vi "Create Wheel Angular Velocity Row_Frame.vi"(7 "use zeros (F)":bool, 8 "error in (no error)":errorcluster, 10 "steering angle (rad)":dbl, 11 "wheel in":refnum<class "NI_Robotics_Wheel.lvclass">) -> (0 "error out":errorcluster, 2 "wheel angular velocity row":dbl[](array[numeric]), 3 "wheel out":refnum<class "NI_Robotics_Wheel.lvclass">)   [LabVIEW 2017, in "NI_Robotics_Wheel.lvclass"]
uses:
  <vilib>/robotics/Steering/Wheel/NI_Robotics_Wheel.lvclass
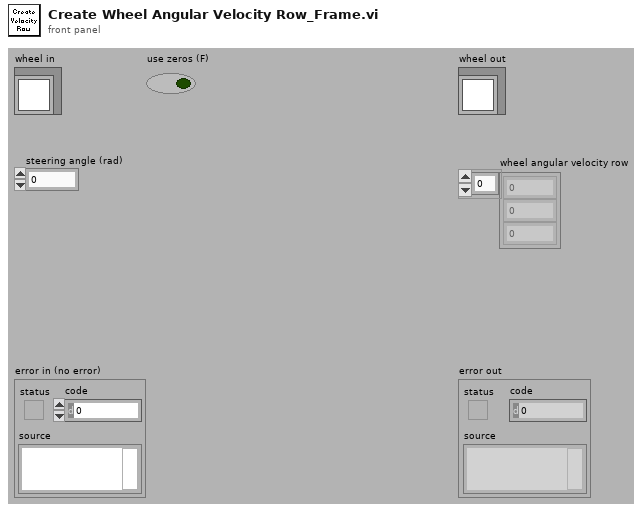
[diagram p1: front panel]
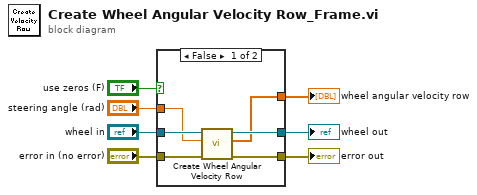
[diagram p0: block diagram]
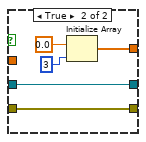
[diagram p2: hidden frame]
diagram:
  n1 = case shown="False" "use zeros (F)" {
    tunnel: "wheel in" -> [w13 w18]
    tunnel: [w12 w18] -> w6
    tunnel: "error in (no error)" -> [w11 w17]
    tunnel: [w10 w17] -> w4
    tunnel: "steering angle (rad)" -> [w9 _]
    tunnel: [w8 w14] -> w2
    frame False {
      n2 = call-dynamic "Create Wheel Angular Velocity Row.vi"("error in (no error)"=w11, "steering angle (rad)"=w9, "wheel in"=w13) -> ("error out"=w10:errorcluster, "wheel angular velocity row"=w8:dbl[], "wheel out"=w12:refnum<class "NI_Robotics_Wheel.lvclass">)  [unwired: 6 in]
    }
    frame True {
      n3 = Initialize Array(0.0, 3 ("dimension size")) -> (w14:dbl[])
    }
  }
  "error out" <- w4
  "wheel out" <- w6
  "wheel angular velocity row" <- w2
